vi "AIT 1553 RT HWOut Loop.vi"() -> ()   [LabVIEW 2013]
uses:
  <vilib>/Platform/TimedLoop/XDataNode/wakeup.ctl
  <vilib>/Platform/TimedLoop/XDataNode/XDNodeRunTimeDep.lvlib
  <vilib>/Platform/TimedLoop/XDataNode/nitl_modes.ctl
  <vilib>/Platform/TimedLoop/XDataNode/timing_clust.ctl
  <vilib>/Platform/TimedLoop/XDataNode/XDataNode.xnode
  RT Controls/ReadWrite Selector.ctl
  AIT 664 Custom Device.lvlib
  RT Controls/AIT 1553 - Bus Section.ctl
  <vilib>/NI Veristand/Custom Device API/Data Reference.ctl
  <vilib>/NI Veristand/Custom Device API/Custom Device API.lvlib
  <vilib>/NI Veristand/Custom Device API/Block Data Reference.ctl
  Controls and Global/Start Bit.ctl
  Controls and Global/Number of Bits.ctl
  RT Controls/FIFO.ctl
  RT Controls/Status Channels Config.ctl
  RT Controls/Label Transfer Config.ctl
  RT Controls/AIT 1553 - Driver Data.ctl
  RT Controls/AIT 664 - RT Message Settings.ctl
  RT Controls/AIT 664 - RT Hardware Channel.ctl
  RT Controls/AIT 664  - RT Data.ctl
  <userlib>/ARINC 664/AIT 664 Controls/General/Direction.ctl
  <userlib>/ARINC 664/AIT 664 API.lvlib
  <userlib>/ARINC 664/AIT 664 Controls/General/Message Port Type.ctl
  <userlib>/ARINC 664/AIT 664 Controls/General/Message Port.ctl
  System Explorer/Controls/664 - Sampling Type.ctl
panel:
  in  "stop":bool
  in  "RT Data":T1 {"End System Handle" format="%x"; "Label Transfer Config"."Block Data Refs"."Data Reference" format="%.0x"; "Status Config"."Hardware Out Dur Reference" format="%.0x"; "Status Config"."Hardware In Dur Reference" format="%.0x"; "Status Config"."Hardware Out Count Reference" format="%.0x"; "Status Config"."Hardware In Count Reference" format="%.0x"; "Status Config"."Error Data Reference" format="%.0x"; "Hardware Output Tx Channels"."Message Settings"."Driver Data"."First Word" min=8 max=31; "Hardware Output Tx Channels"."Message Settings"."Driver Data"."Num Bits" min=1 max=32; "Hardware Output Tx Channels"."Message Settings"."Driver Data"."Start Bit" min=8 max=31; "Hardware Output Tx Channels"."Message Settings"."Block Data Refs"."Data Reference" format="%.0x"; "Hardware Output Tx Channels"."Rx Com Udp Port"."Handle" format="%08x"; "Hardware Output Tx Channels"."Tx Com Udp Port"."Handle" format="%08x"; "Hardware Input Rx Channels"."Message Settings"."Driver Data"."First Word" min=8 max=31; "Hardware Input Rx Channels"."Message Settings"."Driver Data"."Num Bits" min=1 max=32; "Hardware Input Rx Channels"."Message Settings"."Driver Data"."Start Bit" min=8 max=31; "Hardware Input Rx Channels"."Message Settings"."Block Data Refs"."Data Reference" format="%.0x"; "Hardware Input Rx Channels"."Rx Com Udp Port"."Handle" format="%08x"; "Hardware Input Rx Channels"."Tx Com Udp Port"."Handle" format="%08x"}
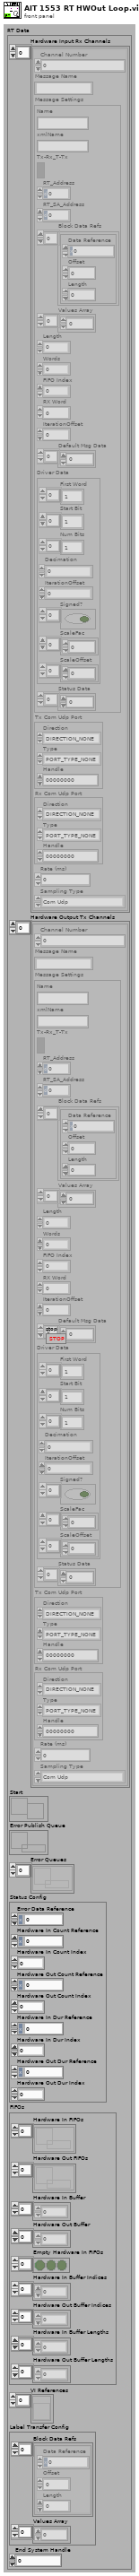
[diagram p1: front panel]
types:
  T1 = typedef "AIT 664 Custom Device.lvlib/AIT 664  - RT Data.ctl" = cluster{"Hardware Input Rx Channels":T2[], "Hardware Output Tx Channels":T2[], "Start":refnum<notifier>, "Error Publish Queue":refnum<queue>, "Error Queues":refnum<queue>[], "Status Config":T13, "FIFOs":T14, "VI References":refnum<vi>[], "Label Transfer Config":T15, "End System Handle ":u64}
  T2 = typedef "AIT 664 Custom Device.lvlib/AIT 664 - RT Hardware Channel.ctl" = cluster{"Channel Number":u16, "Message Name":string, "Message Settings":T3, "Tx Com Udp Port":T9, "Rx Com Udp Port":T9, "Rate (ms)":u32, "Sampling Type":T12}
  T3 = typedef "AIT 664 Custom Device.lvlib/AIT 664 - RT Message Settings.ctl" = cluster{"Name":string, "xmlName":string, "Tx-Rx_T-Tx":bool, "RT_Address":u8, "RT_SA_Address":u8, "Block Data Refs":T4[], "Values Array":dbl[], "Length":i32, "Words":i32, "FIFO Index":i32, "RX Word":u32, "IterationOffset":i32, "Default Msg Data":u8[], "Driver Data":T6, "Status Data":u32[]}
  T4 = typedef "Custom Device API.lvlib/Block Data Reference.ctl" = cluster{"Data Reference":T5, "Offset":i32, "Length":i32}
  T5 = typedef "Custom Device API.lvlib/Data Reference.ctl" = i32
  T6 = typedef "AIT 664 Custom Device.lvlib/AIT 1553 - Driver Data.ctl" = cluster{"First Word":T7[], "Start Bit":T7[], "Num Bits":T8[], "Decimation":i32, "IterationOffset":i32, "Signed?":bool[], "ScaleFac":dbl[], "ScaleOffset":dbl[]}
  T7 = typedef "AIT 664 Custom Device.lvlib/Start Bit.ctl" = i32
  T8 = typedef "AIT 664 Custom Device.lvlib/Number of Bits.ctl" = i32
  T9 = typedef "AIT 664 API.lvlib/Message Port.ctl" = cluster{"Direction":T10, "Type":T11, "Handle":u64}
  T10 = typedef "AIT 664 API.lvlib/Direction.ctl" = enum16{"DIRECTION_NONE", "DIRECTION_TX", "DIRECTION_RX"}
  T11 = typedef "AIT 664 API.lvlib/Message Port Type.ctl" = enum16{"PORT_TYPE_NONE", "COM_UDP", "SAP_UDP", "SAP_IP", "SAP_MAC", "COTS_MAC", "COTS_MAC_RAW"}
  T12 = typedef "AIT 664 Custom Device.lvlib/664 - Sampling Type.ctl" = enum16{"Com Udp", "Com Udp Queuing", "Sap Udp", "Sap Ip", "Sap Mac", "Unknown"}
  T13 = typedef "AIT 664 Custom Device.lvlib/Status Channels Config.ctl" = cluster{"Error Data Reference":T5, "Hardware In Count Reference":T5, "Hardware In Count Index":i32, "Hardware Out Count Reference":T5, "Hardware Out Count Index":i32, "Hardware In Dur Reference":T5, "Hardware In Dur Index":i32, "Hardware Out Dur Reference":T5, "Hardware Out Dur Index":i32}
  T14 = typedef "AIT 664 Custom Device.lvlib/FIFO.ctl" = cluster{"Hardware In FIFOs":refnum<k33>[], "Hardware Out FIFOs":refnum<k33>[], "Hardware In Buffer":dbl[], "Hardware Out Buffer":dbl[], "Empty Hardware In FIFOs":bool[], "Hardware In Buffer Indices":i32[], "Hardware Out Buffer Indices":i32[], "Hardware In Buffer Lengths":i32[], "Hardware Out Buffer Lengths":i32[]}
  T15 = typedef "AIT 664 Custom Device.lvlib/Label Transfer Config.ctl" = cluster{"Block Data Refs":T4[], "Values Array":dbl[]}
  T16 = typedef "AIT 664 Custom Device.lvlib/AIT 1553 - Bus Section.ctl" = enum16{"BC", "BM", "RT"}
  T17 = typedef "AIT 664 Custom Device.lvlib/ReadWrite Selector.ctl" = enum16{"Inline Read", "Inline Write", "Async HWIn", "Async HWOut"}
  T18 = typedef "XDNodeRunTimeDep.lvlib/timing_clust.ctl" = cluster{"Expected End [f-1]":u64, "Actual End [f-1]":u64, "Finished Late? [f-1]":bool, "Expected End [i-1]":u64, "Actual End [i-1]":u64, "Finished Late? [i-1]":bool, "Expected Start [i]":u64, "Actual Start [i]":u64, "Expected Start [f]":u64, "Actual Start [f]":u64, "Source Name":string, "Structure Name":string, "Period":i64, "Deadline":i64, "Offset":i64, "Start":i64, "Priority":i32, "Timeout":i32, "Mode":T19, "Wakeup Reason":T20, "Error":errorcluster, "Source Type":string, "Secondary Source Type":string, "Global End Time":u64, "Global Start Time":u64, "Frame Duration":u64, "Iteration Duration":u64, "Assigned CPU":i32, "I/O Scan Engine Mode":u32}
  T19 = typedef "XDNodeRunTimeDep.lvlib/nitl_modes.ctl" = enum32{"No Change", "Process missed periods, maintain original phase", "Discard missed periods, maintain original phase", "Process missed periods, ignore original phase", "Discard missed periods, ignore original phase"}
  T20 = typedef "XDNodeRunTimeDep.lvlib/wakeup.ctl" = enum32{"Normal", "Aborted", "Asynchronous wakeup", "Timing source error", "Timed loop error", "Timeout"}
  T21 = typedef "AIT 664 Custom Device.lvlib/AIT 664  - RT Data.ctl" = cluster{"Hardware Input Channels":T22[], "Hardware Output Channels":T22[], "Start":refnum<notifier>, "Error Publish Queue":refnum<queue>, "Error Queues":refnum<queue>[], "Status Config":T13, "FIFOs":T14, "VI References":refnum<vi>[], "Label Transfer Config":T15, "End System Handle ":u64}
  T22 = typedef "AIT 664 Custom Device.lvlib/AIT 664 - RT Hardware Channel.ctl" = cluster{"Channel Number":u16, "Message Names":string[], "Message Settings":T3[], "Tx Com Udp Port":T9, "Rx Com Udp Port":T9, "Rate (ms)":u32, "Sampling Type":T12}
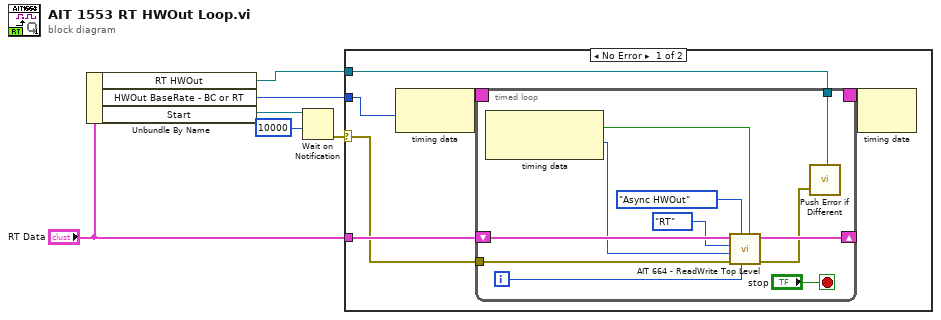
[diagram p0: block diagram]
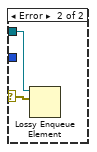
[diagram p2: hidden frame]
diagram:
  n1 = Unbundle By Name("RT Data") -> ("RT HWOut"=w1:refnum<queue>, "HWOut BaseRate - BC or RT"=w6:i64, "Start"=w5:refnum<notifier>)
  n2 = Wait on Notification(notifier=w5, timeout in ms (-1)=10000) -> (error out=w4:errorcluster)  [unwired: 2 in, 3 out]
  n3 = case shown="No Error" w4 {
    selector: w4 -> [w7 w33]
    tunnel: w6 -> [w10 _]
    tunnel: "RT Data" -> [w9 _]
    tunnel: w1 -> [w8 w32]
    frame No Error {
      n4 = node-c288(w10) -> (w12:T18)
      n5 = timed-loop {
        timing: w12 -> [_]
        timing-out: [_] -> w11
        shift-right: [w21] -> _
        shift-left: w9 -> [w22]
        tunnel: w8 -> [w18]
        tunnel: w7 -> [w17]
        i -> [w13]
        stop <- "stop" stop-if-true
        n6 = node-c288() -> (w16:bool, w15:i64)  [unwired: 1 in]
        n7 = call "AIT 664 - ReadWrite Top Level.vi"("Late?"=w16, "Iteration"=w13, "Mode"=ReadWrite_Selector."Async HWOut", "error in (no error)"=w17, "Iteration Duration"=w15, "Bus Section"=AIT_1553_-_Bus_Section."RT", "RT Data in"=w22) -> ("error out"=w19:errorcluster, "RT Data out"=w21:T21)  [unwired: 3 in]
        n8 = call "Push Error if Different.vi"("error in"=w19, "Error Q"=w18) -> ()  [unwired: 1 in]
      }
      n9 = node-c288(w11) -> ()  [unwired: 1 out]
    }
    frame Error {
      n10 = Lossy Enqueue Element(queue=w32, element=w33) -> ()  [unwired: 1 in, 4 out]
    }
  }
